vi "Generate Mock Class.vi"(6 "Add to lvproj?":bool=TRUE, 8 "error in (no error)":errorcluster, 9 "Destination Class Path":path, 10 "Source Class Path":path) -> (0 "error out":errorcluster)   [LabVIEW 2020, in "Mock Class Generator.lvclass"]
uses:
  Mock Class Generator.lvclass
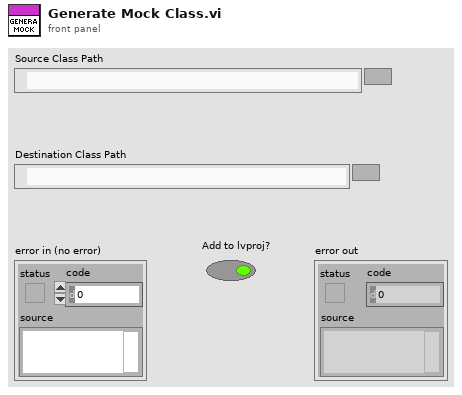
[diagram p1: front panel]
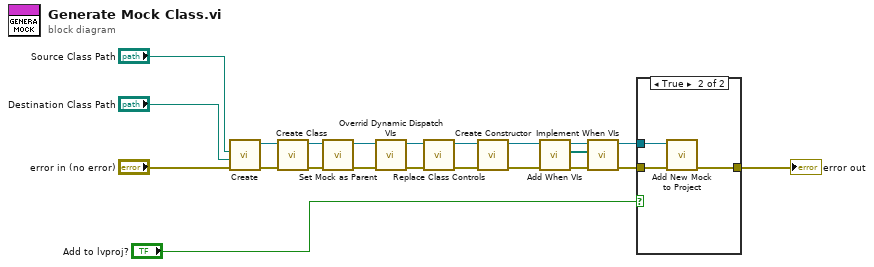
[diagram p0: block diagram]
diagram:
  n1 = call "Create.vi"("error in (no error)"="error in (no error)", "Destination Class Path"="Destination Class Path", "Source Class Path"="Source Class Path") -> ("error out"=w20:errorcluster, "Mock Class Generator Out"=w21:refnum<class "Mock Class Generator.lvclass">)  [unwired: 7 in]
  n2 = call "Create Class.vi"("error in (no error)"=w20, "Mock Class Generator in"=w21) -> ("error out"=w10:errorcluster, "Mock Class Generator out"=w12:refnum<class "Mock Class Generator.lvclass">)  [unwired: 8 in]
  n3 = call "Set Mock as Parent.vi"("error in (no error)"=w10, "Mock Class Generator in"=w12) -> ("error out"=w9:errorcluster, "Mock Class Generator out"=w11:refnum<class "Mock Class Generator.lvclass">)  [unwired: 8 in]
  n4 = call "Overrid Dynamic Dispatch VIs.vi"("error in (no error)"=w9, "Mock Class Generator in"=w11) -> ("error out"=w16:errorcluster, "Mock Class Generator out"=w17:refnum<class "Mock Class Generator.lvclass">)  [unwired: 8 in]
  n5 = call "Replace Class Controls.vi"("error in (no error)"=w16, "Mock Class Generator In"=w17) -> ("error out"=w15:errorcluster, "Mock Class Generator Out"=w13:refnum<class "Mock Class Generator.lvclass">)  [unwired: 8 in]
  n6 = call "Create Constructor.vi"("error in (no error)"=w15, "Mock Class Generator in"=w13) -> ("error out"=w7:errorcluster, "Mock Class Generator"=w6:refnum<class "Mock Class Generator.lvclass">)  [unwired: 8 in]
  n7 = call "Add When VIs.vi"("error in (no error)"=w7, "Mock Class Generator In"=w6) -> ("error out"=w5:errorcluster, "When VIs"=w1:path[], "Mock Class Generator Out"=w3:refnum<class "Mock Class Generator.lvclass">)  [unwired: 7 in]
  n8 = call "Implement When VIs.vi"("error in (no error)"=w5, "When VIs"=w1, "Mock Class Generator In"=w3) -> ("error out"=w4:errorcluster, "Mock Class Generator Out"=w2:refnum<class "Mock Class Generator.lvclass">)  [unwired: 7 in]
  n9 = case shown="True" "Add to lvproj?" {
    tunnel: w4 -> [w23 w26]
    tunnel: [w23 w25] -> w14
    tunnel: w2 -> [_ w24]
    frame False {
    }
    frame True {
      n10 = call "Add New Mock to Project.vi"("error in (no error)"=w26, "Mock Class Generator in"=w24) -> ("error out"=w25:errorcluster)  [unwired: 8 in, 1 out]
    }
  }
  "error out" <- w14
